vi "Debug Window.vi"(4 "Direction":T1, 6 "Action":T2, 7 "Pos":cluster{"Row":i32, "Col":i32}, 9 "Team Idx":i32, 10 "Round":i32, 11 "Hail":refnum<class "Hail.lvclass">) -> ()   [LabVIEW 2015, in "Hail.lvclass"]
uses:
  Hail.lvclass
  Type Defs/Action Enum.ctl
  Type Defs/Direction Enum.ctl
  Hail.lvclass/Hail.ctl
  Type Defs/SB Type Defs.lvlib
panel:
  in  "Continue":bool
  in  "Pause":bool
  in  "Group Stats":i32(listbox)
  in  "Group":i32(listbox)
  in  "Team":i32(listbox)
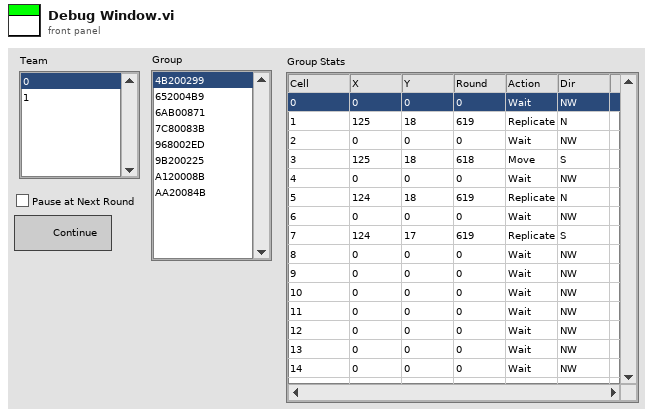
[diagram p1: front panel]
types:
  T1 = typedef "SB Type Defs.lvlib/Direction Enum.ctl" = enum16{"NW", "N", "NE", "E", "SE", "S", "SW", "W"}
  T2 = typedef "SB Type Defs.lvlib/Action Enum.ctl" = enum16{"Wait", "Move", "Attack", "Replicate"}
  T3 = cluster{"DVR[G]":i32[], "Info[G][16]":cluster{"Last Round":i32, "Act":T2, "Dir":T1, "Pos":cluster{"Row":i32, "Col":i32}}[][]}[]
  T4 = cluster{"DVR[G]":i32[], "Info[G][16]":cluster{"Last Round":i32, "Act":T2, "Dir":T1, "Pos":cluster{"Row":i32, "Col":i32}}[][]}
  T5 = cluster{"Last Round":i32, "Act":T2, "Dir":T1, "Pos":cluster{"Row":i32, "Col":i32}}[][]
  T6 = cluster{"Last Round":i32, "Act":T2, "Dir":T1, "Pos":cluster{"Row":i32, "Col":i32}}[]
  T7 = cluster{"Last Round":i32, "Act":T2, "Dir":T1, "Pos":cluster{"Row":i32, "Col":i32}}
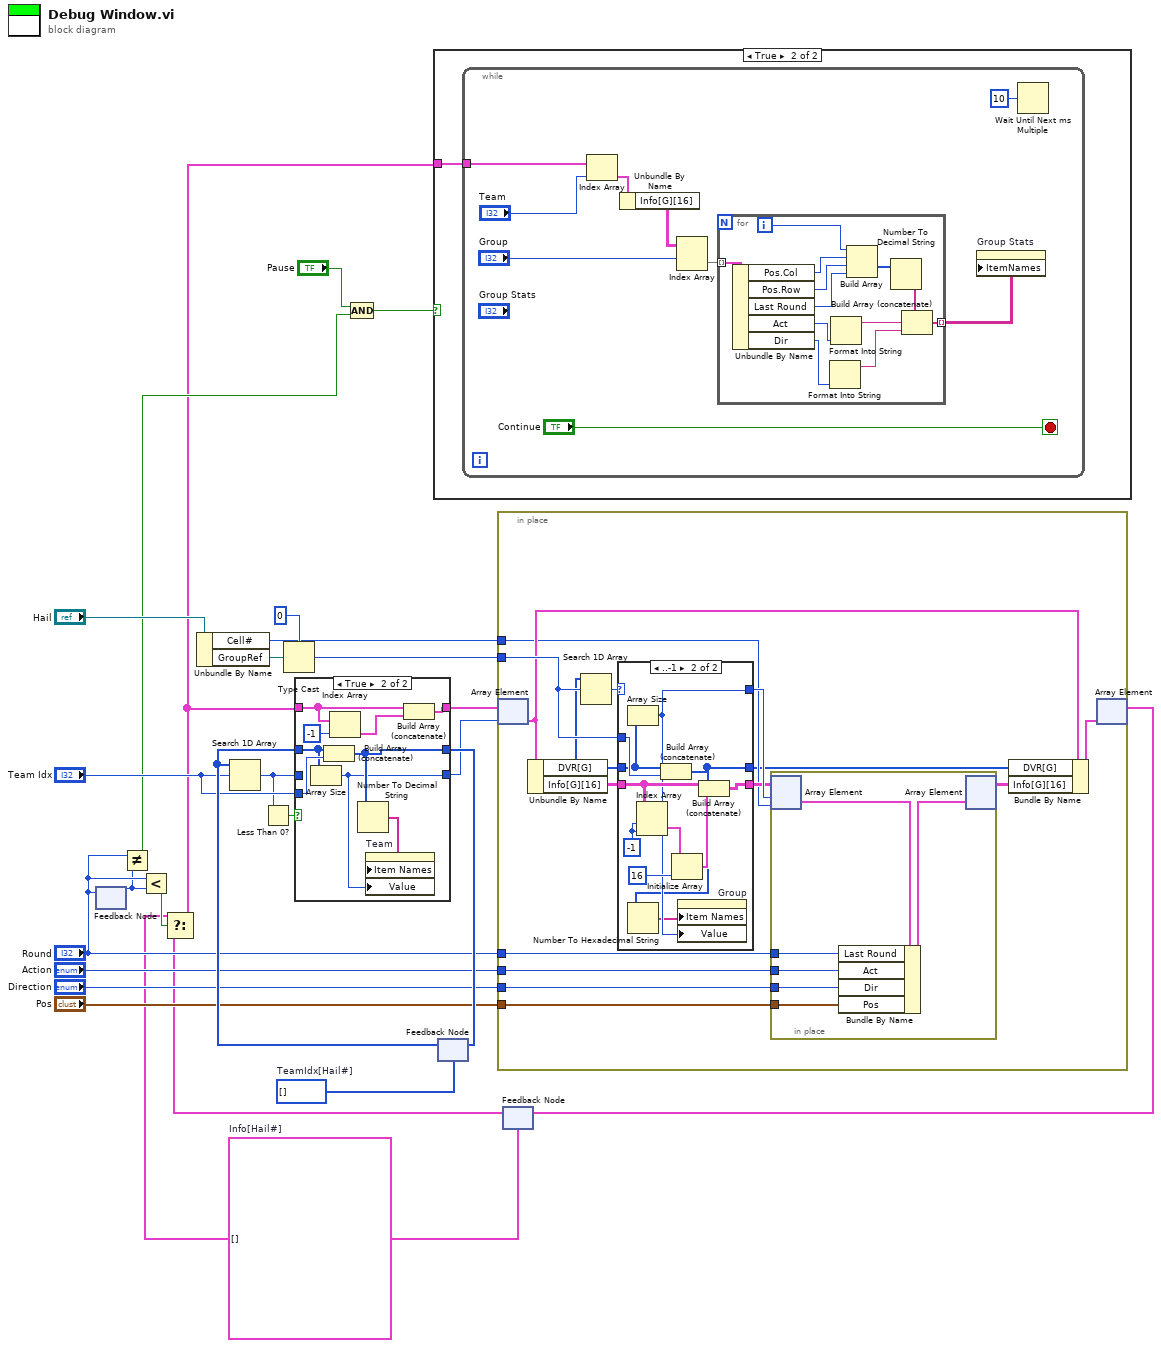
[diagram p0: block diagram]
diagram:
  w1 = T3 []  # Info[Hail#]
  w25 = i32[] []  # TeamIdx[Hail#]
  n1 = feedback #1() -> (w5:i32)  [unwired: 1 in]
  n2 = feedback-in #1("Round") -> ()
  n3 = Not Equal?(x="Round", y=w5) -> (x != y?=w9:bool)
  n4 = Less?(x="Round", y=w5) -> (x < y?=w4:bool)
  n5 = Unbundle By Name("Hail") -> ("Cell#"=w14:i8, "GroupRef"=w19:refnum<data-value>)
  n6 = Type Cast(type=0, x=w19) -> (*(type *) &x=w15:i32)
  n7 = Compound Arithmetic op=AND("Pause", w9) -> (w7:bool)
  n8 = feedback #2(w25) -> (w23:i32[])
  n9 = Search 1D Array(1D array=w23, element="Team Idx") -> (index of element=w21:i32)  [unwired: 1 in]
  n10 = Less Than 0?(x=w21) -> (x < 0?=w24:bool)
  n11 = feedback #3(w1) -> (w3:T3)
  n12 = Select(t=w1, s=w4, f=w3) -> (s? t:f=w2:T3)
  n13 = case shown="True" w24 {
    tunnel: w23 -> [w28 w37]
    tunnel: "Team Idx" -> [_ w38]
    tunnel: w21 -> [w29 _]
    tunnel: [w29 w30] -> w16
    tunnel: [w28 w36] -> w20
    tunnel: w2 -> [w27 w34]
    tunnel: [w27 w31] -> w17
    frame False {
    }
    frame True {
      n14 = Array Size(array=w37) -> (size(s)=w30:i32)
      n15 = Build Array (concatenate)(w37, w38) -> (w36:i32[])
      n16 = Index Array(array=w34, index=-1) -> (element=w32:T4)
      n17 = Number To Decimal String(number=w36) -> (decimal integer string=w35:string[])  [unwired: 1 in]
      n18 = property on="Team" class="LstBox (strict)"("Item Names"=w35, "Value"=w30) -> ()  [unwired: 2 in, 2 out]
      n19 = Build Array (concatenate)(w34, w32) -> (w31:T3)
    }
  }
  n20 = case shown="True" w7 {
    tunnel: w2 -> [_ w39]
    frame False {
    }
    frame True {
      n21 = while {
        tunnel: w39 -> [w47]
        stop <- "Continue" stop-if-true
        n22 = Index Array(array=w47, index="Team") -> (element=w45:T4)
        n23 = Unbundle By Name(w45) -> ("Info[G][16]"=w44:T5)
        n24 = Index Array(array=w44, index (row)="Group") -> (element=w42:T6)  [unwired: 1 in]
        n25 = for {
          tunnel: w42 -> [w60] mode=indexing
          tunnel: [w51] -> w40 mode=indexing
          i -> [w55]
          n26 = Unbundle By Name(w60) -> ("Pos.Col"=w54:i32, "Pos.Row"=w53:i32, "Last Round"=w52:i32, "Act"=w59:T2, "Dir"=w58:T1)
          n27 = Format Into String(w58) -> (resulting string=w56:string)  [unwired: 3 in, 1 out]
          n28 = Format Into String(w59) -> (resulting string=w57:string)  [unwired: 3 in, 1 out]
          n29 = Build Array(w55, w54, w53, w52) -> (w50:i32[])
          n30 = Number To Decimal String(number=w50) -> (decimal integer string=w49:string[])  [unwired: 1 in]
          n31 = Build Array (concatenate)(w49, w57, w56) -> (w51:string[])
        }
        n32 = property on="Group Stats" class="MCListbox (strict)"("ItemNames"=w40) -> ()  [unwired: 2 in, 2 out]
        n33 = Wait Until Next ms Multiple(millisecond multiple=u32 10) -> ()  [unwired: 1 out]
      }
    }
  }
  n34 = feedback-in #2(w20) -> ()
  n35 = in-place {
    in-place-border: w15 -> [w74]
    in-place-border: w14 -> [w67]
    in-place-border: "Round" -> [w64]
    in-place-border: "Action" -> [w63]
    in-place-border: "Direction" -> [w62]
    in-place-border: "Pos" -> [w61]
    n36 = in-place-array #4(w17, w16) -> (w71:T4)
    n37 = Unbundle By Name(w71) -> ("DVR[G]"=w73:i32[], "Info[G][16]"=w72:T5)
    n38 = Search 1D Array(1D array=w73, element=w74) -> (index of element=w75:i32)  [unwired: 1 in]
    n39 = case shown="..-1" w75 {
      selector: w75 -> [w82 _]
      tunnel: w74 -> [_ w95]
      tunnel: w73 -> [w84 w91]
      tunnel: w72 -> [w83 w90]
      tunnel: [w84 w85] -> w65
      tunnel: [w83 w92] -> w68
      tunnel: [w82 w87] -> w69
      frame 0.. {
      }
      frame ..-1 {
        w89 = -1 ("dimension size")
        n40 = Array Size(array=w91) -> (size(s)=w87:i32)
        n41 = Index Array(array=w90, index (row)=w89, index (col)=w89) -> (element=w88:T7)
        n42 = Build Array (concatenate)(w91, w95) -> (w85:i32[])
        n43 = Number To Hexadecimal String(2:w85) -> (0:w86:string[])  [unwired: 1 in]
        n44 = Initialize Array(w88, 16 ("dimension size")) -> (w93:T6)
        n45 = property on="Group" class="LstBox (strict)"("Item Names"=w86, "Value"=w87) -> ()  [unwired: 2 in, 2 out]
        n46 = Build Array (concatenate)(w90, w93) -> (w92:T5)
      }
    }
    n47 = in-place {
      in-place-border: w64 -> [w79]
      in-place-border: w63 -> [w78]
      in-place-border: w62 -> [w77]
      in-place-border: w61 -> [w76]
      n48 = in-place-array #5(w68, w69, w67) -> (w81:T7)
      n49 = Bundle By Name(cluster=w81, "Last Round"=w79, "Act"=w78, "Dir"=w77, "Pos"=w76) -> (w80:T7)
      n50 = in-place-array #5(w80) -> (w66:T5)  [unwired: 2 out]
    }
    n51 = Bundle By Name(cluster=w71, "DVR[G]"=w65, "Info[G][16]"=w66) -> (w70:T4)
    n52 = in-place-array #4(w70) -> (w11:T3)  [unwired: 1 out]
  }
  n53 = feedback-in #3(w11) -> ()
